vi "NaN to Zero array1D.vi"(11 "Array In":dbl[](array[numeric])) -> (3 "Array Out":dbl[](array[numeric]))   [LabVIEW 2016]
panel:
  # "Replace NaNs with zeros in an array"
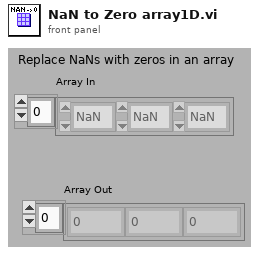
[diagram p1: front panel]
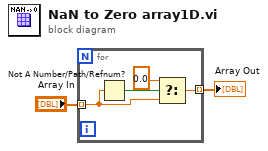
[diagram p0: block diagram]
diagram:
  n1 = for {
    tunnel: "Array In" -> [w5] mode=indexing
    tunnel: [w3] -> w1 mode=indexing
    n2 = Not A Number/Path/Refnum?(number/path/refnum=w5) -> (NaN/Path/Refnum?=w6:bool)
    n3 = Select(t=0.0, s=w6, f=w5) -> (s? t:f=w3:dbl)
  }
  "Array Out" <- w1
